vi "roboRIO v1.0 Build MUX Configuration I2C.vi"(11 "Channel":T4) -> (2 "Configuration Bitmask Array":bool[][](array[boolean]), 3 "Channel Reservation List":T1)   [LabVIEW 2021]
uses:
  <vilib>/myRIO/Common/Instrument Driver Framework/myRIO v1.0/I2C/typedefs/I2C Channels Enum.ctl
  <vilib>/myRIO/Common/Instrument Driver Framework/roboRIO v1.0/Resource Manager/typedefs/roboRIO v1.0 Channel Reservation List.ctl
  <vilib>/myRIO/Common/Instrument Driver Framework/roboRIO v1.0/Resource Manager/typedefs/roboRIO v1.0 Channel Reservation Info.ctl
  <vilib>/myRIO/Common/Instrument Driver Framework/roboRIO v1.0/Resource Manager/typedefs/roboRIO v1.0 Connector List.ctl
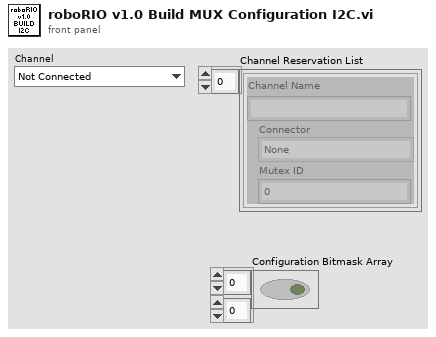
[diagram p1: front panel]
types:
  T1 = typedef "roboRIO v1.0 Channel Reservation List.ctl" = T2[]
  T2 = typedef "roboRIO v1.0 Channel Reservation Info.ctl" = cluster{"Channel Name":string, "Connector":T3, "Mutex ID":i32}
  T3 = typedef "roboRIO v1.0 Connector List.ctl" = enum32{"None", "ConnectorB", "ConnectorI2C", "ConnectorDIO", "ConnectorRSL", "ConnectorRELAY", "ConnectorAI", "ConnectorPWM", "ConnectorSPI"}
  T4 = typedef "I2C Channels Enum.ctl" = enum16{"Not Connected", "A/I2C", "B/I2C", "I2C/I2C"}
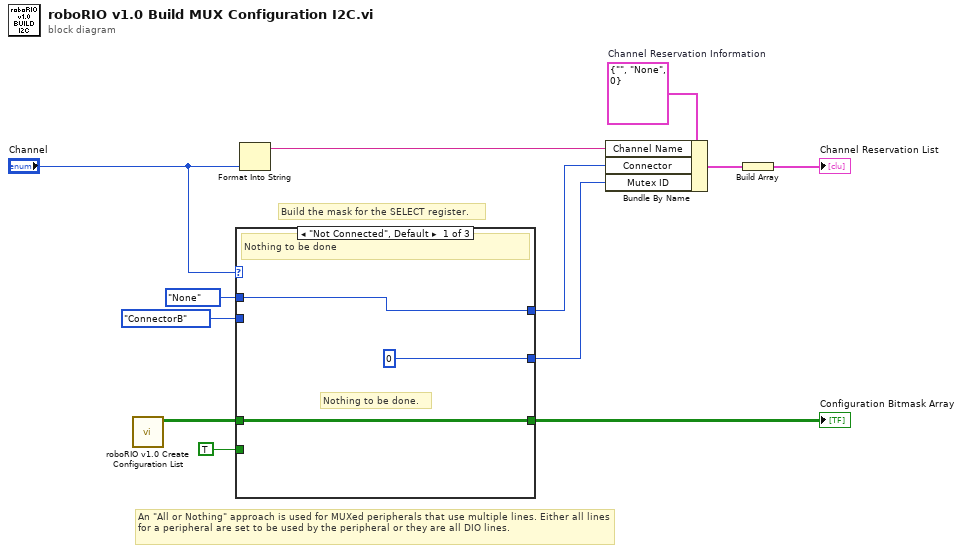
[diagram p0: block diagram]
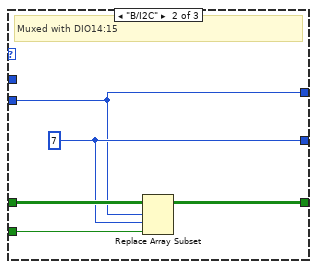
[diagram p2: hidden frame]
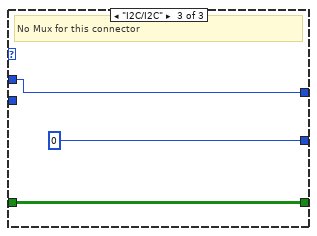
[diagram p3: hidden frame]
diagram:
  w5 = T2 {"Channel Name"="", "Connector"=enum."None", "Mutex ID"=0}  # Channel Reservation Information
  # "An \"All or Nothing\" approach is used for MUXed peripherals that use multiple lines. Either all lines for a peripheral are set to be used by the peripheral or they are all DIO lines."
  # "Build the mask for the SELECT register."
  n1 = call <vilib>:"roboRIO v1.0 Create Configuration List.vi"() -> ("Bitmask Array"=w3:bool[][])  [unwired: 11 in]
  n2 = case shown="\"Not Connected\", Default" "Channel" {
    tunnel: w3 -> [w15 w20 w22]
    tunnel: [w15 w19 w22] -> w9
    tunnel: roboRIO_v1.0_Connector_List."None" ("Connector List") -> [w14 _ w21]
    tunnel: roboRIO_v1.0_Connector_List."ConnectorB" ("Connector List") -> [_ w16 _]
    tunnel: TRUE ("new element/subarray") -> [_ w18 _]
    tunnel: [0 ("index") w17 0 ("index")] -> w7
    tunnel: [w14 w16 w21] -> w8
    frame "Not Connected", Default {
      # "Nothing to be done."
      # "Nothing to be done"
    }
    frame "B/I2C" {
      w17 = 7 ("index")
      # "Muxed with DIO14:15"
      n3 = Replace Array Subset(array=w20, new element=w18, index (row)=w16, index (col)=w17) -> (w19:bool[][])
    }
    frame "I2C/I2C" {
      # "No Mux for this connector"
    }
  }
  "Configuration Bitmask Array" <- w9
  n4 = Format Into String("Channel") -> (resulting string=w4:string)  [unwired: 3 in, 1 out]
  n5 = Bundle By Name(cluster=w5, "Channel Name"=w4, "Connector"=w8, "Mutex ID"=w7) -> (w2:T2)
  n6 = Build Array(w2) -> (→"Channel Reservation List":T2[])
